vi "CleanUp.vi"(0 "object in":refnum<class "PrepareKickoffAllyPlayVSS.lvclass">, 5 "error in (no error)":errorcluster) -> (14 "object out":refnum<class "PrepareKickoffAllyPlayVSS.lvclass">, 19 "error out":errorcluster)   [LabVIEW 2023, in "PrepareKickoffAllyPlayVSS.lvclass"]
uses:
  PrepareKickoffAllyPlayVSS.lvclass
  Play_class/Play.lvclass
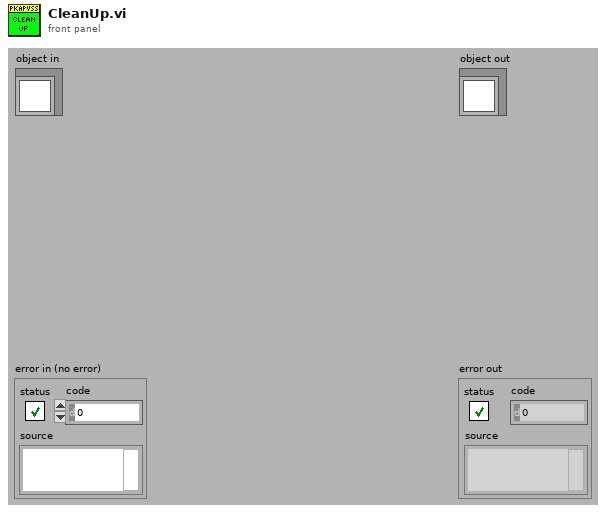
[diagram p1: front panel]
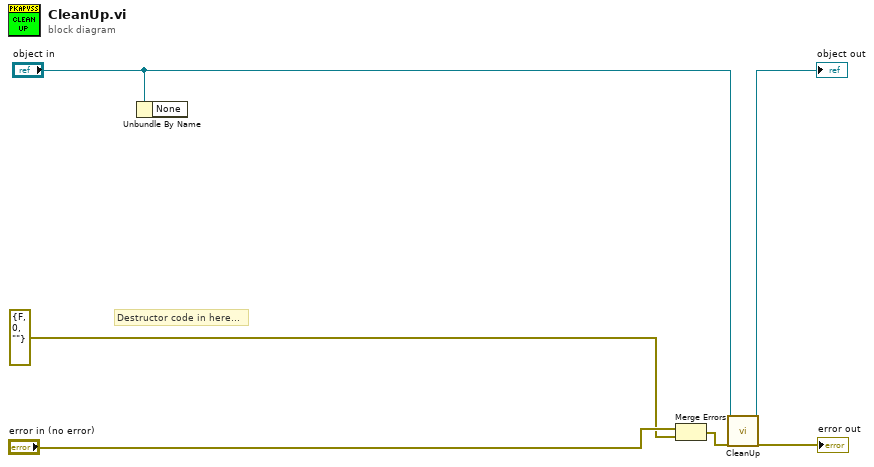
[diagram p0: block diagram]
diagram:
  # "Destructor code in here..."
  n1 = Unbundle By Name("object in") -> ()  [unwired: 1 out]
  n2 = Merge Errors("error in (no error)", errorcluster {"status"=FALSE, "code"=0, "source"=""} ("error in (no error)")) -> (w4:errorcluster)
  n3 = call-parent "CleanUp.vi"("object in"="object in", "error in (no error)"=w4) -> ("object out"=→"object out":refnum<class "PrepareKickoffAllyPlayVSS.lvclass">, "error out"=→"error out":errorcluster)  [unwired: 16 in]
